vi "FGV_MovRel_Values.vi"(8 "error in":errorcluster, 10 "Action":T1, 11 "MovRel position IN":dbl[](array[numeric])) -> (0 "error out":errorcluster, 3 "MovRel position array OUT":dbl[](array[numeric]))   [LabVIEW 2026]
doc: "Functional Global Variable:\n- Write the value into the memory \nor\n- Read the value from the memory"
uses:
  TypeDef_FGV.ctl
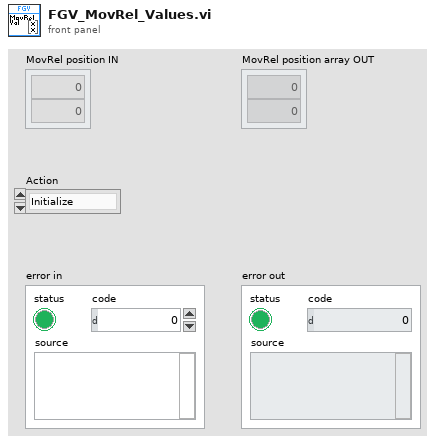
[diagram p1: front panel]
types:
  T1 = typedef "TypeDef_FGV.ctl" = enum16{"Initialize", "Write", "Read"}
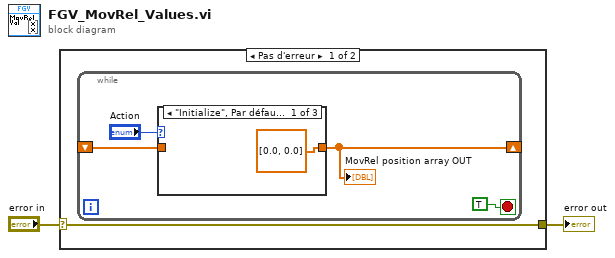
[diagram p0: block diagram]
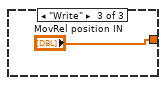
[diagram p3: hidden frame]
diagram:
  n1 = case shown="Pas d'erreur" "error in" {
    selector: "error in" -> [w3 w11]
    tunnel: [w3 w11] -> w1
    frame No Error {
      n2 = while {
        shift-right: [w4] -> _
        shift-left: _ -> [w5]
        stop <- TRUE stop-if-true
        n3 = case shown="\"Initialize\", Par défaut" "Action" {
          tunnel: w5 -> [_ w9 _]
          tunnel: [dbl[] [0.0, 0.0] w9 "MovRel position IN"] -> w4
          frame "Initialize", Default {
          }
          frame "Read" {
          }
          frame "Write" {
          }
        }
        "MovRel position array OUT" <- w4
      }
    }
    frame Error {
    }
  }
  "error out" <- w1
